vi "set home settings.vi"(8 "error in (no error)":errorcluster, 10 "home_settings":T1, 11 "id":i32) -> (0 "error out":errorcluster, 3 "function return":i32)   [LabVIEW 2012, in "libximc.lvlib"]
doc: "result_t XIMC_API set_home_settings (device_t id, const home_settings_t* home_settings);"
uses:
  libximc.lvlib
  libximc.dll
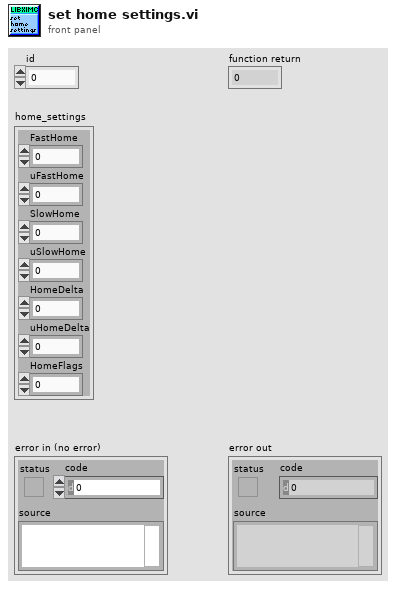
[diagram p1: front panel]
types:
  T1 = cluster{"FastHome":u32, "uFastHome":u32, "SlowHome":u32, "uSlowHome":u32, "HomeDelta":i32, "uHomeDelta":i32, "HomeFlags":u32}
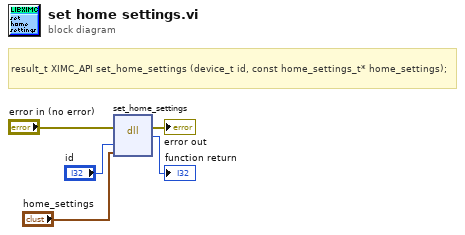
[diagram p0: block diagram]
diagram:
  # "result_t XIMC_API set_home_settings (device_t id, const home_settings_t* home_settings);"
  n1 = dll-call lib="E:/labview-2.12.1-Labview_12.0/ximcLVx32/libximc.*" fn="set_home_settings"(error in="error in (no error)", "id"="id", "home_settings"="home_settings") -> (error out=→"error out":errorcluster, →"function return":i32)  [unwired: 4 in, 1 out]
